vi "Test Program.vi"() -> ()   [LabVIEW 2018, in "VICI M50.lvlib"]
uses:
  VICI M50/VICI M50.lvlib
  Settings Cluster.ctl
  VICI M6 M50 Party Mode.lvlib
panel:
  out "Connection Error":bool
  out "Pump On?":enum16{"Off", "On", "Not Initialized"}(ring)
  in  "stop":bool
  in  "Pause":bool
  in  "speed":dbl
  out "error in (no error) 2":errorcluster
  in  "error in (no error)":errorcluster
  out "VICI Settings 2":T1={"VISA resource name"="", "Simulated?"=TRUE, "Pump Letter"="", "Reverse?"=FALSE}
  in  "VICI Settings":T1={"VISA resource name"="", "Simulated?"=TRUE, "Pump Letter"="", "Reverse?"=FALSE}
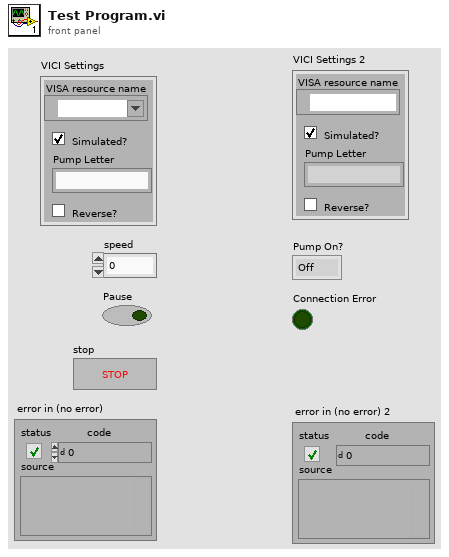
[diagram p1: front panel]
types:
  T1 = typedef "VICI M6 M50 Party Mode.lvlib/Settings Cluster.ctl" = cluster{"VISA resource name":refnum<visa-resource-name>, "Simulated?":bool, "Pump Letter":string, "Reverse?":bool}
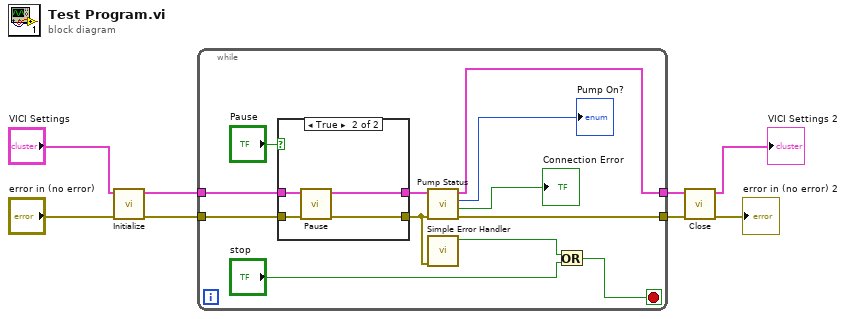
[diagram p0: block diagram]
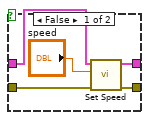
[diagram p2: hidden frame]
diagram:
  n1 = call "Initialize.vi"("error in (no error)"="error in (no error)", "VICI Settings"="VICI Settings") -> ("error out"=w1:errorcluster, "VICI Settings"=w2:T1)  [unwired: 6 in, 2 out]
  n2 = while {
    tunnel: [w20] -> w4
    tunnel: [w19] -> w3
    tunnel: w2 -> [w17]
    tunnel: w1 -> [w16]
    stop <- w12 stop-if-true
    n3 = case shown="True" "Pause" {
      tunnel: [w22 w29] -> w18
      tunnel: [w23 w28] -> w9
      tunnel: w17 -> [w25 w27]
      tunnel: w16 -> [w24 w26]
      frame False {
        n4 = call "Set Speed.vi"("error in (no error)"=w24, "speed"="speed", "VICI Settings"=w25) -> ("error out"=w23:errorcluster, "VICI Settings"=w22:T1)  [unwired: 6 in, 1 out]
      }
      frame True {
        n5 = call "Pause.vi"("error in (no error)"=w26, "VICI Settings"=w27) -> ("error out"=w28:errorcluster, "VICI Settings"=w29:T1)  [unwired: 8 in]
      }
    }
    n6 = call "Pump Status.vi"("error in (no error)"=w9, "VICI Settings"=w18) -> ("error out"=w19:errorcluster, "Connection Error"=→"Connection Error":bool, "Pump On?"=→"Pump On?":enum16{"Off", "On", "Not Initialized"}, "VICI Settings"=w20:T1)  [unwired: 6 in]
    n7 = call <vilib>:"Simple Error Handler.vi"("error in (no error)"=w9) -> ("error?"=w11:bool)  [unwired: 4 in, 4 out]
    n8 = Or(x=w11, y="stop") -> (x .or. y?=w12:bool)
  }
  n9 = call "Close.vi"("error in (no error)"=w3, "VICI Settings"=w4) -> ("error out"=→"error in (no error) 2":errorcluster, "VICI Settings"=→"VICI Settings 2":T1)  [unwired: 8 in]
